vi "Data To SingleElementsArray.vi"(6 "Separator(/)":string="/", 8 "error in (no error)":errorcluster, 10 "parentUrl":string, 11 "Cluster":variant) -> (0 "error out":errorcluster, 1 "Tree Description":string[][](array[string]), 2 "Full NameList":string[](array[string]), 3 "DataElementArray":variant[](array[variant]))   [LabVIEW 2017]
doc: "Flattens a cluster into an array of its individual elements, naming each by its path below parentUrl joined with Seperator. The flat name list and a two-dimensional tree description are returned as well."
uses:
  <vilib>/Utility/Data Type/NI_Data Type.lvlib
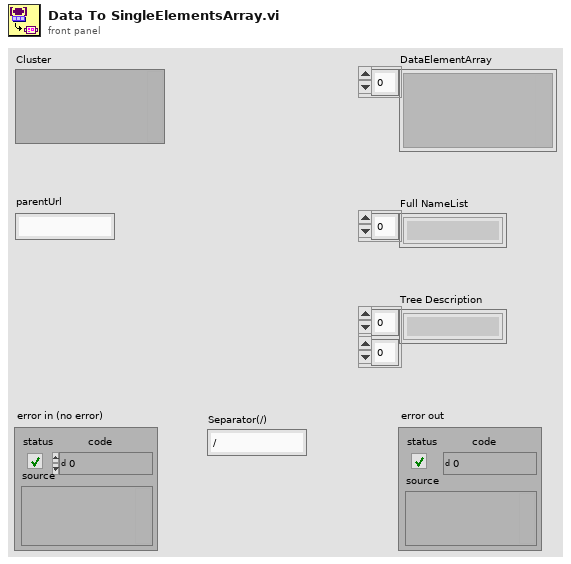
[diagram p1: front panel]
types:
  T1 = typedef "NI_Data Type.lvlib/Data Type.ctl" = enum8{"Invalid Type", "Void", "I8", "I16", "I32", "I64", "U8", "U16", "U32", "U64", "Single Float", "Double Float", "Extended Float", "Single Complex", "Double Complex", "Extended Complex", "Enum U8", "Enum U16", "Enum U32", "Enum U64", "Single Float With Unit", "Double Float With Unit", "Extended Float With Unit", "Single Complex with Unit", "Double Complex with Unit", "Extended Complex with Unit", "Boolean", "String", "Path", "Picture", "Tag", "Array", "Cluster", "Variant", "LV Variant", "Waveform", "Timestamp", "Digital Waveform", "Digital Data", "ExpressData", "Refnum", "External Data", "VI", "Poly VI", "LabVIEW Class Instance", "Fixed Point"}
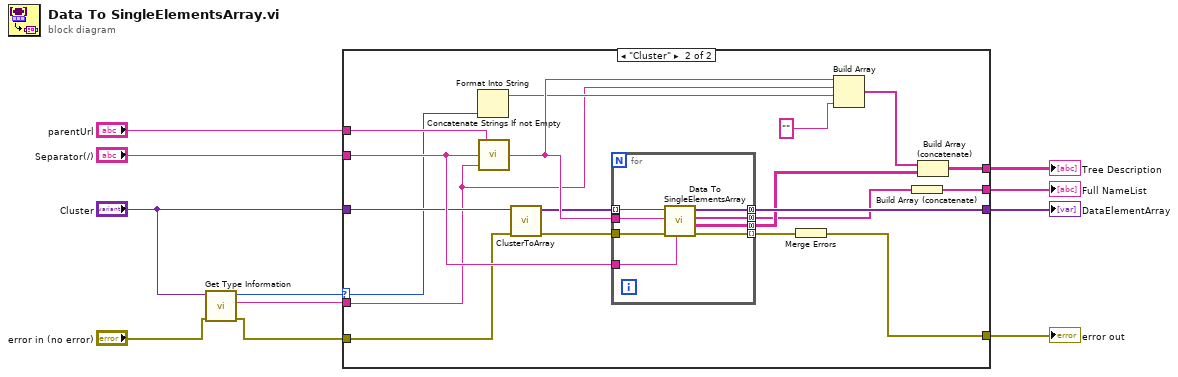
[diagram p0: block diagram]
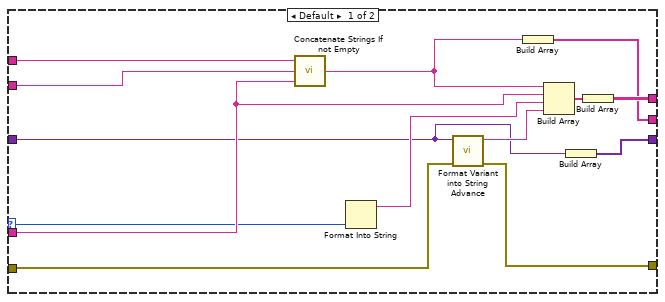
[diagram p2: hidden frame]
diagram:
  n1 = call <vilib>:"Get Type Information.vi"("error in (no error)"="error in (no error)", "Variant"="Cluster") -> ("error out"=w2:errorcluster, "Name"=w1:string, "Type"=w4:T1)  [unwired: 5 in, 2 out]
  n2 = case shown="\"Cluster\"" w4 {
    selector: w4 -> [w12 w26]
    tunnel: "Cluster" -> [w14 w29]
    tunnel: "parentUrl" -> [w25 w42]
    tunnel: [w20 w40] -> w8
    tunnel: w2 -> [w13 w28]
    tunnel: [w22 w43] -> w10
    tunnel: [w21 w36] -> w9
    tunnel: [w18 w33] -> w7
    tunnel: "Separator(/)" -> [w16 w30]
    tunnel: w1 -> [w15 w27]
    frame Default {
      n3 = call "Concatenate Strings If not Empty.vi"("String"=w15, "seperator(:)"=w16, "prefix"=w25) -> ("result"=w19:string)  [unwired: 2 in]
      n4 = Format Into String(w12) -> (resulting string=w17:string)  [unwired: 3 in, 1 out]
      n5 = call "Format Variant into String Advance.vi"("error in (no error)"=w13, "Variant"=w14) -> ("error out"=w22:errorcluster, "Data"=w24:string)  [unwired: 7 in, 1 out]
      n6 = Build Array(w19) -> (w18:string[])
      n7 = Build Array(w19, w15, w17, w24) -> (w23:string[])
      n8 = Build Array(w14) -> (w21:variant[])
      n9 = Build Array(w23) -> (w20:string[][])
    }
    frame "Cluster" {
      n10 = Format Into String(w26) -> (resulting string=w32:string)  [unwired: 3 in, 1 out]
      n11 = call "Concatenate Strings If not Empty.vi"("String"=w27, "seperator(:)"=w30, "prefix"=w42) -> ("result"=w38:string)  [unwired: 2 in]
      n12 = call "ClusterToArray.vi"("Error in"=w28, "Cluster"=w29) -> ("Error out"=w31:errorcluster, "Array"=w37:variant[])  [unwired: 8 in]
      n13 = for {
        tunnel: w37 -> [w52] mode=indexing
        tunnel: w38 -> [w51]
        tunnel: [w50] -> w36 mode=concatenating
        tunnel: w31 -> [w49]
        tunnel: [w48] -> w44 mode=indexing
        tunnel: [w47] -> w35 mode=concatenating
        tunnel: [w46] -> w34 mode=concatenating
        tunnel: w30 -> [w45]
        n14 = call "Data To SingleElementsArray.vi"("Separator(/)"=w45, "error in (no error)"=w49, "parentUrl"=w51, "Cluster"=w52) -> ("error out"=w48:errorcluster, "Tree Description"=w47:string[][], "Full NameList"=w46:string[], "DataElementArray"=w50:variant[])  [unwired: 4 in]
      }
      n15 = Merge Errors(w44) -> (w43:errorcluster)
      n16 = Build Array(w38, w27, w32, "" ("element")) -> (w39:string[])
      n17 = Build Array (concatenate)(w34) -> (w33:string[])
      n18 = Build Array (concatenate)(w39, w35) -> (w40:string[][])
    }
  }
  "Full NameList" <- w7
  "error out" <- w10
  "DataElementArray" <- w9
  "Tree Description" <- w8
